vi "GetInfo.vi"(8 "Error In":errorcluster, 11 "reference in":refnum<class "Circle.lvclass">) -> (0 "Error Out":errorcluster, 2 "Console":string, 3 "reference out":refnum<class "Circle.lvclass">)   [LabVIEW 2020, in "Circle.lvclass"]
uses:
  Circle.lvclass
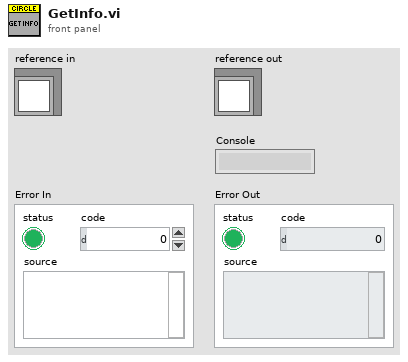
[diagram p1: front panel]
types:
  T1 = typedef "Circle.lvclass/ObjectAttributes.ctl" = cluster{"_radius":i32}
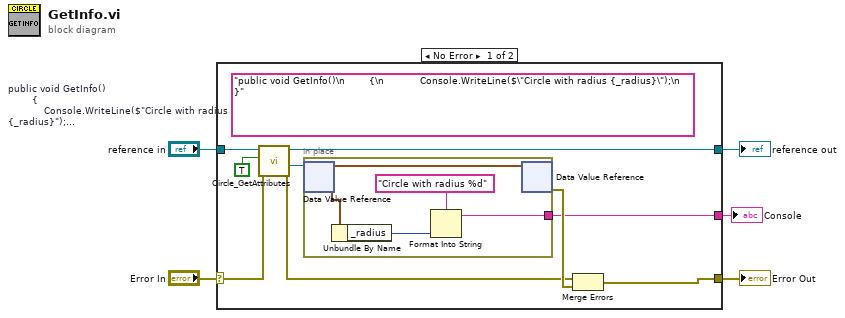
[diagram p0: block diagram]
diagram:
  n1 = case shown="No Error" "Error In" {
    selector: "Error In" -> [w13 w20]
    tunnel: [w10 w20] -> w4
    tunnel: [w11 w19] -> w2
    tunnel: "reference in" -> [w14 w19]
    tunnel: [w6 _] -> w1
    frame No Error {
      (unwired) "public void GetInfo()\n        {\n            Console.WriteLine($\"Circle with radius {_radius}\");\n        }"  # public void GetInfo()         {             Console.WriteLine($"Circle with radius {_radius}");         }
      n2 = call "Circle_GetAttributes.vi"("error in (no error)"=w13, "OnlyGetDvrReference(False)"=TRUE, "reference in"=w14) -> ("error out"=w8:errorcluster, "DataRef"=w9:refnum<data-value>, "reference out"=w11:refnum<class "Circle.lvclass">)  [unwired: 5 in, 1 out]
      n3 = in-place {
        in-place-border: [w16] -> w6
        n4 = in-place-dvr #1(w9) -> (w15:T1)  [unwired: 1 out]
        n5 = Unbundle By Name(w15) -> ("_radius"=w18:i32)
        n6 = Format Into String(format string="Circle with radius %d", w18) -> (resulting string=w16:string)  [unwired: 2 in, 1 out]
        n7 = in-place-dvr #1(w15) -> (w12:errorcluster)  [unwired: 1 out]
      }
      n8 = Merge Errors(w8, w12) -> (w10:errorcluster)
    }
    frame Error {
    }
  }
  "Error Out" <- w4
  "reference out" <- w2
  "Console" <- w1
